vi "Write Club Number.vi"(8 "error in (no error)":errorcluster, 10 "Club Number":i32, 11 "Golf Club in":refnum<class "Golf Club.lvclass">) -> (0 "error out":errorcluster, 3 "Golf Club out":refnum<class "Golf Club.lvclass">)   [LabVIEW 2019, in "Golf Club.lvclass"]
uses:
  Golf Club.lvclass
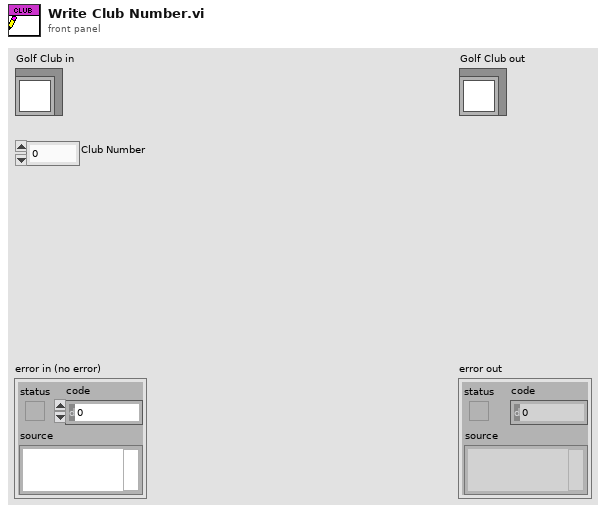
[diagram p1: front panel]
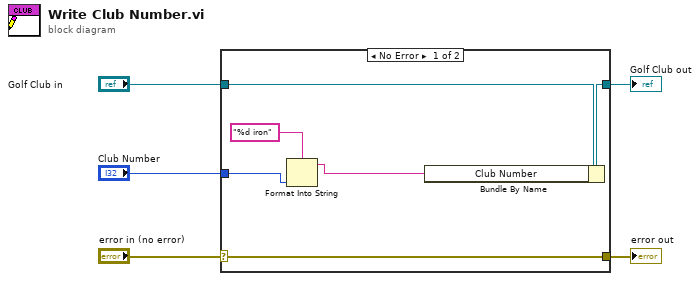
[diagram p0: block diagram]
diagram:
  n1 = case shown="No Error" "error in (no error)" {
    selector: "error in (no error)" -> [w11 w12]
    tunnel: [w11 w12] -> w4
    tunnel: [w9 w13] -> w2
    tunnel: "Golf Club in" -> [w10 w13]
    tunnel: "Club Number" -> [w8 _]
    frame No Error {
      n2 = Format Into String(format string="%d iron", w8) -> (resulting string=w6:string)  [unwired: 2 in, 1 out]
      n3 = Bundle By Name(cluster=w10, "Club Number"=w6) -> (w9:refnum<class "Golf Club.lvclass">)
    }
    frame Error {
    }
  }
  "error out" <- w4
  "Golf Club out" <- w2
